vi "NanotecSMCPDDriver.set limit switch props.vi"(0 "VISA resource name":refnum<visa-resource-name>, 1 "contollerID":i32=-1, 3 "limitSwitchProperties (17442)":bool[](array[boolean])=[FALSE, TRUE, FALSE, FALSE, FALSE, TRUE, FALSE, FALSE, FALSE, FALSE, TRUE, FALSE, FALSE, FALSE, TRUE, FALSE], 5 "error in (no error)":errorcluster) -> (14 "VISA resource name out":refnum<visa-resource-name>, 15 "contollerID out":i32=-1, 19 "error out":errorcluster)   [LabVIEW 2014, in "NanotecSMCPDDriver.lvlib"]
doc: "Sets the properties for the limit switches. This VI should only be used by experts during the commisisioning phase."
uses:
  NanotecSMCPDDriver.lvlib
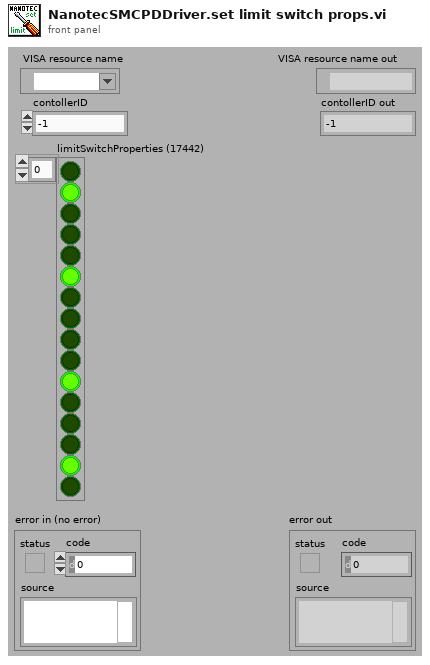
[diagram p1: front panel]
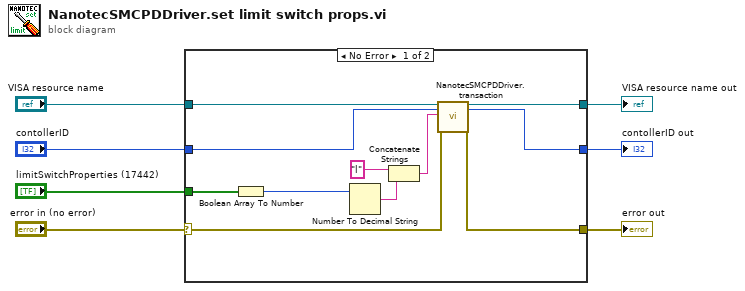
[diagram p0: block diagram]
diagram:
  n1 = case shown="No Error" "error in (no error)" {
    selector: "error in (no error)" -> [w13 w19]
    tunnel: [w15 w21] -> w7
    tunnel: [w14 w19] -> w6
    tunnel: "VISA resource name" -> [w18 w21]
    tunnel: "contollerID" -> [w17 w20]
    tunnel: [w16 w20] -> w3
    tunnel: "limitSwitchProperties (17442)" -> [w8 _]
    frame No Error {
      n2 = Boolean Array To Number(Boolean array=w8) -> (number=w9:u32)
      n3 = Number To Decimal String(number=w9) -> (decimal integer string=w12:string)  [unwired: 1 in]
      n4 = Concatenate Strings("l" ("commandString"), w12) -> (w10:string)
      n5 = call "NanotecSMCPDDriver.transaction.vi"("VISAresource"=w18, "contollerID"=w17, "commandString"=w10, "error in (no error)"=w13) -> ("VISAresource out"=w15:refnum<visa-resource-name>, "contollerID out"=w16:i32, "error out"=w14:errorcluster)  [unwired: 10 in, 3 out]
    }
    frame Error {
    }
  }
  "VISA resource name out" <- w7
  "error out" <- w6
  "contollerID out" <- w3
